vi "BigDataFits_I16_FGV.vi"(8 "InError":errorcluster caption="entrée d'erreur (pas d'erreur)", 9 "ClustBigFilFits":T1={"file (use dialog)"=path "D:/DATA/Imatest.fits", "Type de données"=enum."I16 (signed integer 16bit)", "Commentaire"="", "naxis1"=0, "naxis2"=0, "naxis3"=1, "Exptime"=1.0}, 10 "entier 16 bits":i16[][](array[numeric]), 11 "Énum":T3) -> (0 "sortie d'erreur":errorcluster)   [LabVIEW 2020]
uses:
  BigDataFits.ctl
  ClustBigFilFits.ctl
  DataTyp_Header.ctl
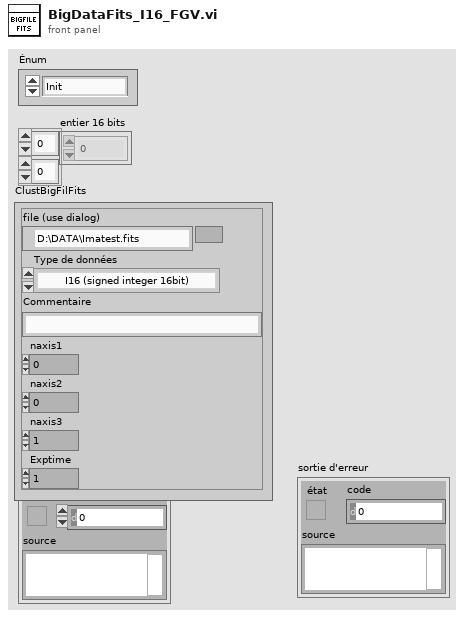
[diagram p1: front panel]
types:
  T1 = typedef "ClustBigFilFits.ctl" = cluster{"file (use dialog)":path, "Type de données":T2, "Commentaire":string, "naxis1":i32, "naxis2":i32, "naxis3":i32, "Exptime":sgl}
  T2 = typedef "DataTyp_Header.ctl" = enum16{"U8 (unsigned integer 8bit)", "I16 (signed integer 16bit)", "U16 (unsigned integer 16 bit)", "I32 (signed integer 32bit)", "U32 (unsigned integer 32 bit)", "SGL (float 32bit)", "DBL(float 64bit)", "complex (2xfloat 64bit)"}
  T3 = typedef "BigDataFits.ctl" = enum16{"Init", "WritHeader", "WritData", "Close"}
  T4 = enum16{"open", "replace", "create", "open or create", "replace or create", "replace or create with confirmation"}
  T5 = enum16{"big-endian, network order", "native, host order", "little-endian"}
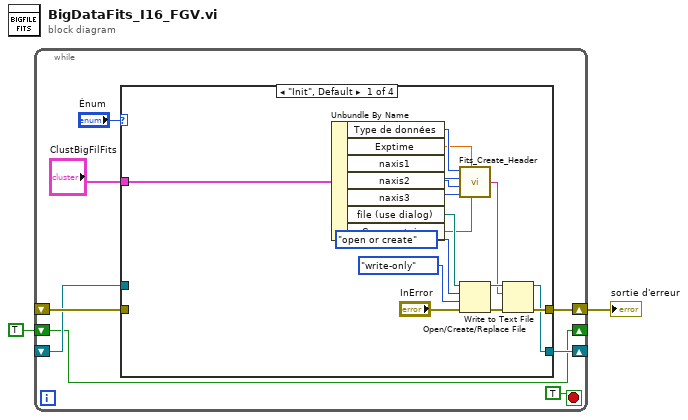
[diagram p0: block diagram]
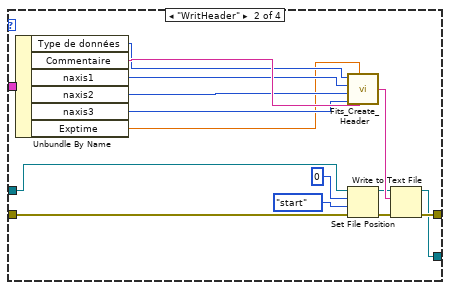
[diagram p2: hidden frame]
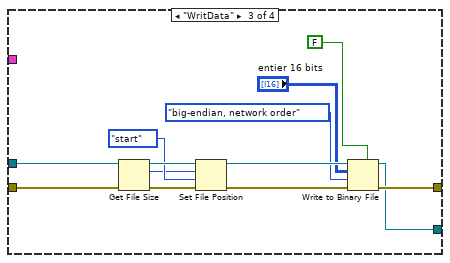
[diagram p3: hidden frame]
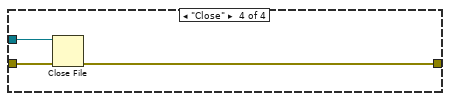
[diagram p4: hidden frame]
diagram:
  n1 = while {
    shift-right: [w4] -> _
    shift-left: TRUE -> [w4]
    shift-right: [w7] -> _
    shift-left: _ -> [w5]
    shift-right: [w8] -> w2
    shift-left: _ -> [w6]
    stop <- TRUE stop-if-true
    n2 = case shown="\"Init\", Default" "Énum" {
      tunnel: [w20 w41 w45 w57] -> w8
      tunnel: [w19 w40 w44 _] -> w7
      tunnel: w6 -> [_ w36 w47 w58]
      tunnel: w5 -> [_ w35 w46 w56]
      tunnel: "ClustBigFilFits" -> [w18 w33 _ _]
      frame "Init", Default {
        n3 = Unbundle By Name(w18) -> ("Type de données"=w13:T2, "Exptime"=w11:sgl, "naxis1"=w16:i32, "naxis2"=w15:i32, "naxis3"=w14:i32, "file (use dialog)"=w17:path, "Commentaire"=w12:string)
        n4 = call "Fits_Create_Header.vi"("Commentaire"=w12, "Exptim"=w11, "naxis3"=w14, "naxis2"=w15, "naxis1"=w16, "Type de données"=w13) -> ("FITS header"=w21:string)
        n5 = Open/Create/Replace File(file path (use dialog)=w17, error in="InError", operation (0:open)=T4."open or create" ("opération (0 : open)"), access (0:read/write)=enum16{"read/write", "read-only", "write-only"}."write-only" ("accès (0 : read/write)")) -> (refnum out=w22:refnum<file>, error out=w23:errorcluster)  [unwired: 2 in, 1 out]
        n6 = Write to Text File(file (use dialog)=w22, text=w21, error in=w23) -> (refnum out=w19:refnum<file>, error out=w20:errorcluster)  [unwired: 1 in, 1 out]
      }
      frame "WritHeader" {
        n7 = Unbundle By Name(w33) -> ("Type de données"=w28:T2, "Commentaire"=w32:string, "naxis1"=w29:i32, "naxis2"=w30:i32, "naxis3"=w31:i32, "Exptime"=w27:sgl)
        n8 = call "Fits_Create_Header.vi"("Commentaire"=w32, "Exptim"=w27, "naxis3"=w31, "naxis2"=w30, "naxis1"=w29, "Type de données"=w28) -> ("FITS header"=w42:string)
        n9 = Set File Position(offset (in bytes) (0)=i64 0 ("offset (en octets) (0)"), refnum=w35, from (0:start)=enum16{"start", "end", "current"}."start" ("à partir de (0 : start)"), error in=w36) -> (refnum out=w34:refnum<file>, error out=w37:errorcluster)
        n10 = Write to Text File(file (use dialog)=w34, text=w42, error in=w37) -> (refnum out=w40:refnum<file>, error out=w41:errorcluster)  [unwired: 1 in, 1 out]
      }
      frame "WritData" {
        n11 = Get File Size(file=w46, error in=w47) -> (refnum out=w55:refnum<file>, size (in bytes)=w52:i64, 0:w53:errorcluster)
        n12 = Set File Position(offset (in bytes) (0)=w52, refnum=w55, from (0:start)=enum16{"start", "end", "current"}."start" ("à partir de (0 : start)"), error in=w53) -> (refnum out=w50:refnum<file>, error out=w51:errorcluster)
        n13 = Write to Binary File(file (use dialog)=w50, data="entier 16 bits", error in=w51, 5:FALSE ("ajouter une taille de tableau ou de chaîne ? (V)"), 9:T5."big-endian, network order" ("ordre des octets (0 : big-Endian, network order)")) -> (refnum out=w44:refnum<file>, error out=w45:errorcluster)  [unwired: 1 in, 1 out]
      }
      frame "Close" {
        n14 = Close File(refnum=w56, error in=w58) -> (error out=w57:errorcluster)  [unwired: 1 out]
      }
    }
  }
  "sortie d'erreur" <- w2
